vi "Create Test Configuration.vi"() -> (0 "error out":errorcluster, 1 "Names":string[](array[string]), 2 "File Name":string, 3 "Module Configuration":refnum<class "SystemLink File configuration.lvclass">, 4 "Folder Path":path, 5 "instance identifier":string, 6 "Channels":refnum<class "TBM channel.lvclass">[](array[class]))   [LabVIEW 2015, in "SystemLink File Module tests.lvlib"]
doc: "This VI creates a standard test configuration for other unit tests. It currently creates and adds one line with every datatype to the module configuration."
uses:
  SystemLink File Module tests.lvlib
  module/configuration/SystemLink File configuration.lvclass
  <vilib>/NI/Tag Bus Module Framework/channel/TBM channel.lvclass
  module/configuration/Connection Type.ctl
  module/configuration/Connection Configuration.ctl
  <vilib>/NI/Tag Bus/tag/Data Type.ctl
  <vilib>/NI/Tag Bus Module Framework/channel/channel classification.ctl
  module/configuration/SystemLink File configuration.lvclass/SystemLink File configuration.ctl
  <vilib>/NI/Tag Bus/tag/tag descriptor.lvclass/tag descriptor.ctl
  module/configuration/Write Connection Configuration.vi
  <vilib>/NI/Configuration Framework/serializable configuration/NISE_CEF_serializable configuration.lvclass
  <vilib>/NI/Tag Bus/tag/tag descriptor.lvclass
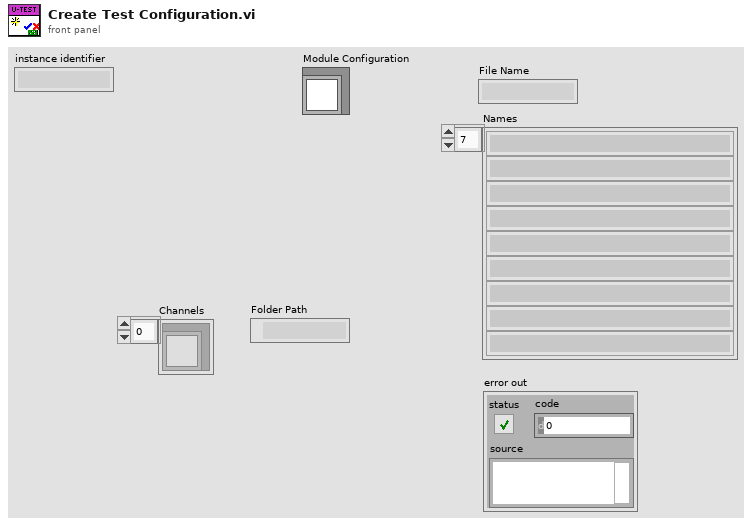
[diagram p1: front panel]
types:
  T1 = typedef "TBM channel.lvclass/channel classification.ctl" = enum16{"input data", "output data", "processing parameter", "processing result"}
  T2 = typedef "tag bus.lvlib/tag descriptor.lvclass/Data Type.ctl" = enum16{"Double", "Single", "I64", "I32", "I16", "I8", "U64", "U32", "U16", "U8", "Boolean", "String", "Array of Double", "Array of Single", "Array of I64", "Array of I32", "Array of I16", "Array of I8", "Array of U64", "Array of U32", "Array of U16", "Array of U8", "Array of Boolean", "Array of String"}
  T3 = typedef "SystemLink File configuration.lvclass/Connection Configuration.ctl" = cluster{"Connection Type":T4, "AMQP":cluster{"Configuration ID":string}, "HTTP":cluster{"Verify Server?":bool, "Server URL":string, "CA Certificate File":string, "User Info":cluster{"Username":string, "Password":string}, "API Key":string}}
  T4 = typedef "SystemLink File configuration.lvclass/Connection Type.ctl" = enum16{"AMQP", "HTTP", "API Key (SystemLink Cloud)"}
  T5 = cluster{"Verify Server?":bool, "Server URL":string, "CA Certificate File":string, "User Info":cluster{"Username":string, "Password":string}, "API Key":string}
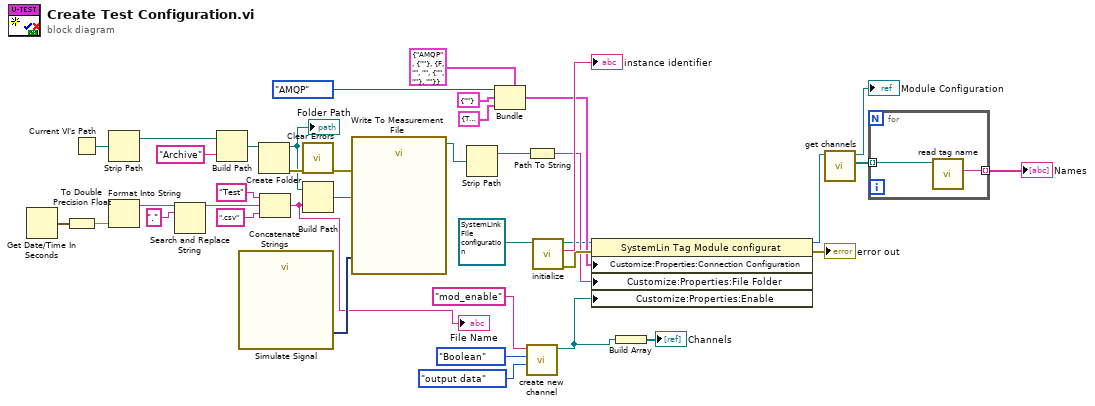
[diagram p0: block diagram]
diagram:
  n1 = Get Date/Time In Seconds() -> (seconds since 1Jan1904=w7:timestamp)
  n2 = To Double Precision Float(number=w7) -> (double precision float=w8:dbl)
  n3 = Current VI's Path() -> (path=w18:path)
  n4 = Strip Path(path=w18) -> (stripped path=w17:path)  [unwired: 1 out]
  n5 = Format Into String(w8) -> (resulting string=w6:string)  [unwired: 3 in, 1 out]
  n6 = Search and Replace String(input string=w6, search string=".") -> (result string=w4:string)  [unwired: 6 in, 3 out]
  n7 = Build Path(base path=w17, name or relative path="Archive") -> (appended path=w13:path)
  n8 = call "Simulate Signal"() -> ("Sine"=w26:dynamicdata)  [unwired: 14 in, 1 out]
  n9 = Create Folder(path (use dialog)=w13) -> (created path=w9:path, error out=w12:errorcluster)  [unwired: 2 in, 1 out]
  "Folder Path" <- w9
  n10 = Concatenate Strings("Test" ("name or relative path"), w4, ".csv" ("string")) -> (w3:string)
  "File Name" <- w3
  n11 = call <vilib>:"Clear Errors.vi"("error in (no error)"=w12) -> ("error out"=w11:errorcluster)  [unwired: 5 in, 1 out]
  n12 = Build Path(base path=w9, name or relative path=w3) -> (appended path=w10:path)
  n13 = call "Write To Measurement File"("Signals"=w26, "error in (no error)"=w11, "Filename"=w10) -> ("Filename Out"=w20:path)  [unwired: 14 in, 2 out]
  n14 = Strip Path(path=w20) -> (stripped path=w19:path)  [unwired: 1 out]
  n15 = Bundle(cluster=T3 {"Connection Type"=enum."AMQP", "AMQP"={"Configuration ID"=""}, "HTTP"={"Verify Server?"=FALSE, "Server URL"="", "CA Certificate File"="", "User Info"={"Username"="", "Password"=""}, "API Key"=""}} ("Connection Configuration"), "Connection Type"=Connection_Type."AMQP", "AMQP"=cluster{"Configuration ID":string} {"Configuration ID"=""}, "HTTP"=T5 {"Verify Server?"=TRUE, "Server URL"="Server URL", "CA Certificate File"="\\ni-rt\\system", "User Info"={"Username"="username", "Password"="password"}, "API Key"="API Key"}) -> (w31:T3)
  n16 = Path To String(path=w19) -> (string=w30:string)
  n17 = call <vilib>:"create new channel.vi"("channel classification"=channel_classification."output data", "data type"=Data_Type."Boolean", "channel name"="mod_enable") -> ("channel"=w2:refnum<class "TBM channel.lvclass">)  [unwired: 8 in]
  n18 = call <vilib>:"initialize.vi"("configuration in"=refnum<class "SystemLink File configuration.lvclass"> refnum ("tag bus configurable plugin module configuration")) -> ("error out"=w38:errorcluster, "identifier"=→"instance identifier":string, "configuration out"=w29:refnum<class "SystemLink File configuration.lvclass">)  [unwired: 8 in]
  n19 = property class="SystemLin Tag Module configurat"(reference=w29, error in=w38, "Customize:Properties:Connection Configuration"=w31, "Customize:Properties:File Folder"=w30, "Customize:Properties:Enable"=w2) -> (reference out=w22:refnum<class "SystemLink File configuration.lvclass">, error out=→"error out":errorcluster)
  n20 = Build Array(w2) -> (→"Channels":refnum<class "TBM channel.lvclass">[])
  n21 = call-dynamic "get channels.vi"("SystemLin Tag Module configuration in"=w22) -> ("channels"=w27:refnum<class "TBM channel.lvclass">[], "SystemLin Tag Module configuration out"=→"Module Configuration":refnum<class "SystemLink File configuration.lvclass">)  [unwired: 9 in]
  n22 = for {
    tunnel: w27 -> [w41] mode=indexing
    tunnel: [w40] -> w28 mode=indexing
    n23 = call <vilib>:"read tag name.vi"("system tag in"=w41) -> ("name"=w40:string)  [unwired: 8 in, 2 out]
  }
  "Names" <- w28
